vi "Unescape String.vi"(11 "Escaped String":string) -> (3 "String":string)   [LabVIEW 2020, in "JSON.lvlib"]
uses:
  JSON.lvlib
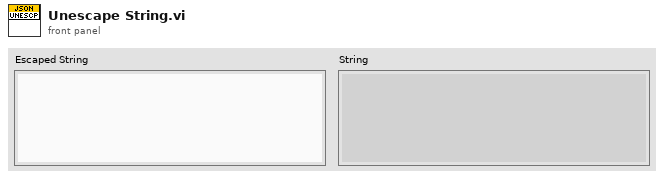
[diagram p1: front panel]
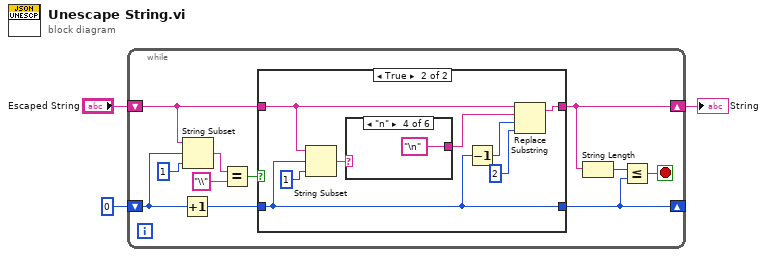
[diagram p0: block diagram]
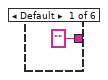
[diagram p3: hidden frame]
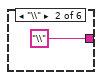
[diagram p4: hidden frame]
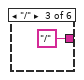
[diagram p5: hidden frame]
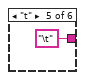
[diagram p6: hidden frame]
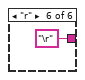
[diagram p7: hidden frame]
diagram:
  n1 = while {
    shift-right: [w8] -> w1
    shift-left: "Escaped String" -> [w10]
    shift-right: [w4] -> _
    shift-left: 0 -> [w13]
    stop <- w6 stop-if-true
    n2 = Increment(x=w13) -> (x+1=w9:i32)
    n3 = String Subset(string=w10, offset (0)=w13, length (rest)=1 ("length (rest)")) -> (substring=w5:string)
    n4 = Equal?(x=w5, y="\\") -> (x = y?=w11:bool)
    n5 = case shown="True" w11 {
      tunnel: w10 -> [w16 w21]
      tunnel: w9 -> [w15 w18]
      tunnel: [w15 w18] -> w4
      tunnel: [w16 w20] -> w8
      frame False {
      }
      frame True {
        n6 = String Subset(string=w21, offset (0)=w18, length (rest)=1 ("length (rest)")) -> (substring=w23:string)
        n7 = case shown="\"n\"" w23 {
          tunnel: ["" ("substring (\"\")") "\\" ("substring (\"\")") "/" ("substring (\"\")") "\n" ("substring (\"\")") "\t" ("substring (\"\")") "\r" ("substring (\"\")")] -> w19
          frame Default {
          }
          frame "\\" {
          }
          frame "/" {
          }
          frame "n" {
          }
          frame "t" {
          }
          frame "r" {
          }
        }
        n8 = Decrement(x=w18) -> (x-1=w17:i32)
        n9 = Replace Substring(2:2 ("y"), 3:w17, 4:w19, 5:w21) -> (1:w20:string)  [unwired: 1 out]
      }
    }
    n10 = String Length(string=w8) -> (length=w7:i32)
    n11 = Less Or Equal?(x=w7, y=w4) -> (x <= y?=w6:bool)
  }
  "String" <- w1
